vi "ReversedEngineering HideClassMethods.vi"(1 "Item Paths":path[](array[path]), 5 "error in (no error)":errorcluster) -> (15 "Item Paths filtered":path[](array[path]), 19 "error out":errorcluster)   [LabVIEW 2012]
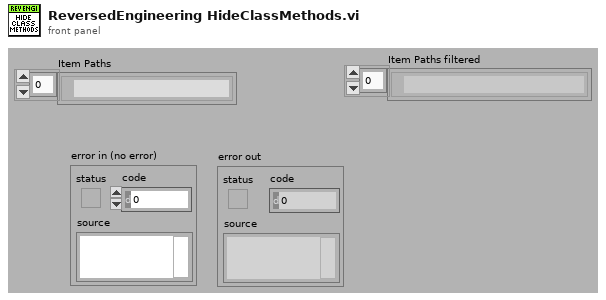
[diagram p1: front panel]
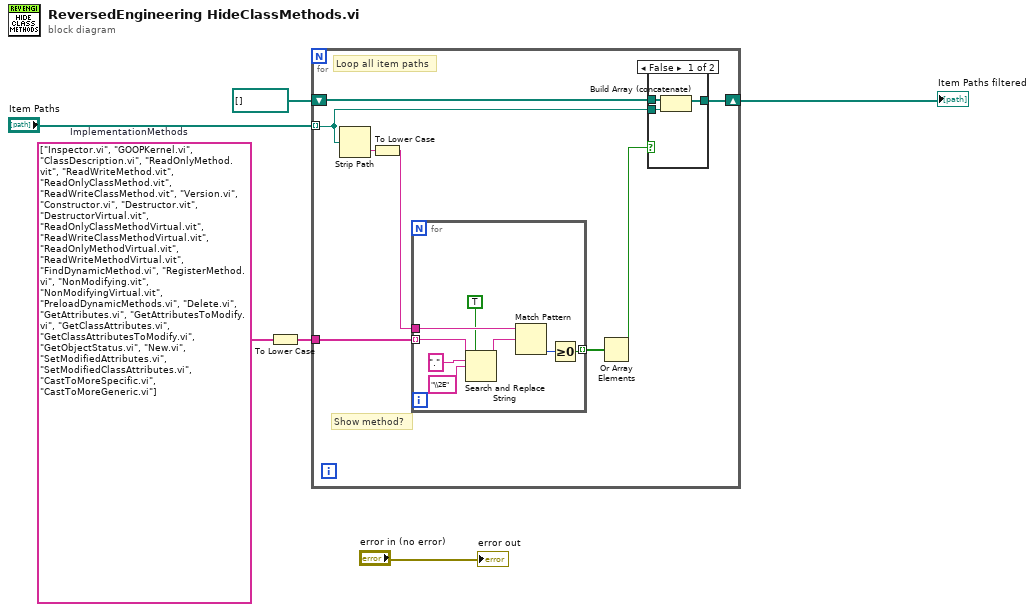
[diagram p0: block diagram]
diagram:
  w2 = string[] ["Inspector.vi", "GOOPKernel.vi", "ClassDescription.vi", "ReadOnlyMethod.vit", "ReadWriteMethod.vit", "ReadOnlyClassMethod.vit", "ReadWriteClassMethod.vit", "Version.vi", "Constructor.vi", "Destructor.vit", "DestructorVirtual.vit", "ReadOnlyClassMethodVirtual.vit", "ReadWriteClassMethodVirtual.vit", "ReadOnlyMethodVirtual.vit", "ReadWriteMethodVirtual.vit", "FindDynamicMethod.vi", "RegisterMethod.vi", "NonModifying.vit", "NonModifyingVirtual.vit", "PreloadDynamicMethods.vi", "Delete.vi", "GetAttributes.vi", "GetAttributesToModify.vi", "GetClassAttributes.vi", "GetClassAttributesToModify.vi", "GetObjectStatus.vi", "New.vi", "SetModifiedAttributes.vi", "SetModifiedClassAttributes.vi", "CastToMoreSpecific.vi", "CastToMoreGeneric.vi"]  # ImplementationMethods
  n1 = To Lower Case(string=w2) -> (all lower case string=w3:string[])
  n2 = for {
    tunnel: "Item Paths" -> [w14] mode=indexing
    shift-right: [w12] -> w5
    shift-left: path[] [] -> [w13]
    tunnel: w3 -> [w7]
    # "Show method?"
    # "Loop all item paths"
    n3 = Strip Path(path=w14) -> (name=w11:string)  [unwired: 1 out]
    n4 = To Lower Case(string=w11) -> (all lower case string=w10:string)
    n5 = for {
      tunnel: w7 -> [w19] mode=indexing
      tunnel: w10 -> [w22]
      tunnel: [w20] -> w9 mode=indexing
      n6 = Search and Replace String(replace all?=TRUE ("replace all? (F)"), input string=w19, search string=".", replace string="\\2E" ("replace string (\"\")")) -> (result string=w18:string)  [unwired: 1 in, 6 out]
      n7 = Match Pattern(string=w22, regular expression=w18) -> (offset past match=w21:i32)  [unwired: 4 out]
      n8 = Greater Or Equal To 0?(x=w21) -> (x >= 0?=w20:bool)
    }
    n9 = Or Array Elements(Boolean array=w9) -> (logical OR=w8:bool)
    n10 = case shown="False" w8 {
      tunnel: w14 -> [w25 _]
      tunnel: w13 -> [w24 w26]
      tunnel: [w23 w26] -> w12
      frame False {
        n11 = Build Array (concatenate)(w24, w25) -> (w23:path[])
      }
      frame True {
      }
    }
  }
  "Item Paths filtered" <- w5
  "error out" <- "error in (no error)"
